vi "ExtractData2.vi"(8 "Samples per freq calc":dbl=10000.0, 11 "Data input":waveform(dbl)[](array[waveform])) -> ()   [LabVIEW 2019]
uses:
  <vilib>/measure/NI_MAPro.lvlib
  <vilib>/measure/madcrms.llb/Basic Averaged DC-RMS for 1 Chan.vi
  <vilib>/gmath/NI_Gmath.lvlib
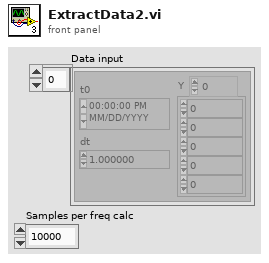
[diagram p1: front panel]
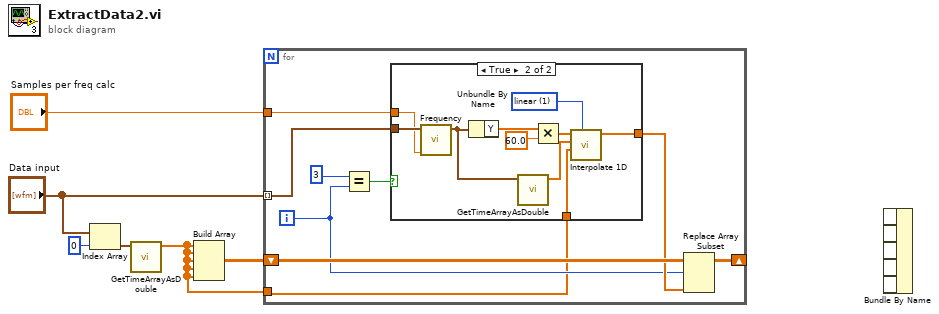
[diagram p0: block diagram]
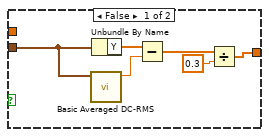
[diagram p2: hidden frame]
diagram:
  n1 = Index Array(array="Data input", index=0) -> (element=w6:waveform(dbl))
  n2 = call "GetTimeArrayAsDouble.vi"("Waveform"=w6) -> ("Time Array"=w1:dbl[])  [unwired: 10 in]
  n3 = Build Array(w1, w1, w1, w1, w1) -> (w2:dbl[][])
  n4 = for {
    tunnel: "Data input" -> [w14] mode=indexing
    tunnel: "Samples per freq calc" -> [w12]
    shift-right: [w11] -> _
    shift-left: w2 -> [w10]
    tunnel: w1 -> [w7]
    i -> [w8]
    n5 = Equal?(x=3, y=w8) -> (x = y?=w15:bool)
    n6 = case shown="True" w15 {
      tunnel: [w16 w24] -> w9
      tunnel: w14 -> [w21 w31]
      tunnel: w12 -> [_ w22]
      tunnel: w7 -> [_ w27]
      frame False {
        n7 = call-poly <vilib>:"Basic Averaged DC-RMS.vi"("signal in"=w21) -> ("DC value"=w17:dbl)  [unwired: 7 in, 3 out]
        n8 = Unbundle By Name(w21) -> ("Y"=w18:dbl[])
        n9 = Subtract(x=w18, y=w17) -> (x-y=w19:dbl[])
        n10 = Divide(x=w19, y=0.3) -> (x/y=w16:dbl[])
      }
      frame True {
        w23 = 1 items=["nearest", "linear", "spline", "cubic Hermite", "Lagrange"] ("method")
        n11 = call "Frequency.vi"("Samples per calculation"=w22, "Input waveform"=w31) -> ("Frequency waveform"=w25:waveform(dbl))  [unwired: 9 in]
        n12 = Unbundle By Name(w25) -> ("Y"=w30:dbl[])
        n13 = call "GetTimeArrayAsDouble.vi"("Waveform"=w25) -> ("Time Array"=w26:dbl[])  [unwired: 10 in]
        n14 = Multiply(x=w30, y=60.0) -> (x*y=w28:dbl[])
        n15 = call <vilib>:"Interpolate 1D.vi"("method"=w23, "xi"=w27, "X"=w26, "Y"=w28) -> ("yi"=w24:dbl[])  [unwired: 5 in, 2 out]
      }
    }
    n16 = Replace Array Subset(array=w10, new element=w9, index (row)=w8) -> (w11:dbl[][])  [unwired: 1 in]
  }
  n17 = Bundle By Name() -> ()  [unwired: 6 in, 1 out]
